vi "Read Stop Disk Action.vi"(8 "error in (no error)":errorcluster, 11 "File Worker in":refnum<class "File Worker.lvclass">) -> (0 "error out":errorcluster, 2 "Stop Disk Action":refnum<notifier>, 3 "File Worker out":refnum<class "File Worker.lvclass">)   [LabVIEW 2025, in "File Worker.lvlib" / "File Worker.lvclass"]
uses:
  File Worker.lvclass
  File Worker.lvclass/File Worker.ctl
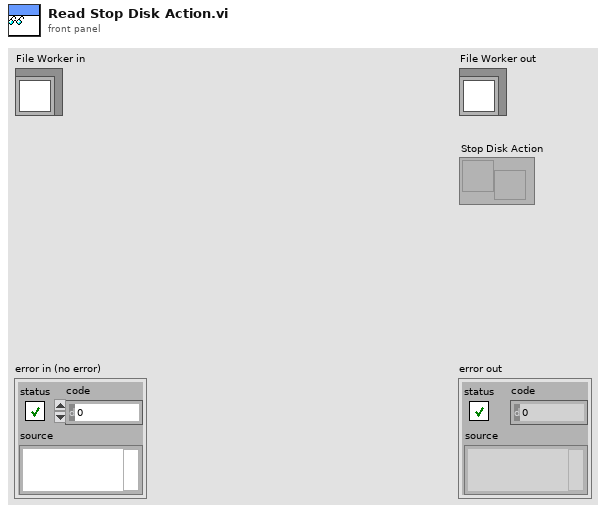
[diagram p1: front panel]
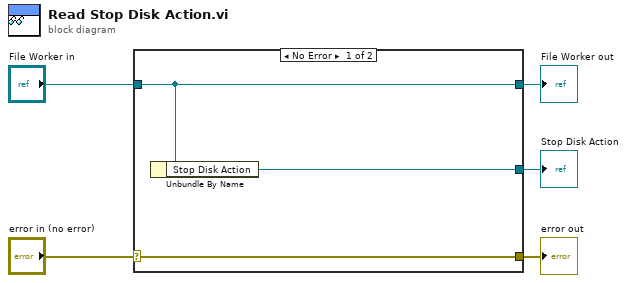
[diagram p0: block diagram]
diagram:
  n1 = case shown="No Error" "error in (no error)" {
    selector: "error in (no error)" -> [w8 w9]
    tunnel: [w8 w9] -> w4
    tunnel: [w7 w10] -> w2
    tunnel: "File Worker in" -> [w7 w10]
    tunnel: [w6 _] -> w1
    frame No Error {
      n2 = Unbundle By Name(w7) -> ("Stop Disk Action"=w6:refnum<notifier>)
    }
    frame Error {
    }
  }
  "error out" <- w4
  "File Worker out" <- w2
  "Stop Disk Action" <- w1
